vi "in_delta values.vi"(11 "x array":dbl[](array[numeric])) -> (3 "x delta values":dbl[](array[numeric]))   [LabVIEW 2020, in "NI_Gmath.lvlib"]
uses:
  NI_Gmath.lvlib
  NI_AALPro.lvlib
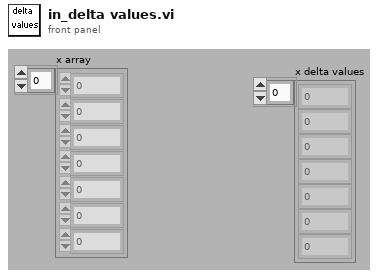
[diagram p1: front panel]
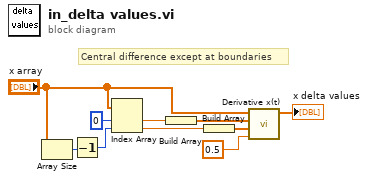
[diagram p0: block diagram]
diagram:
  # "Central difference except at boundaries"
  n1 = Array Size(array="x array") -> (size(s)=w10:i32)
  n2 = Decrement(x=w10) -> (x-1=w8:i32)
  n3 = Index Array(array="x array", index #1=0 ("index"), index #2=w8) -> (element #1=w7:dbl, element #2=w5:dbl)
  n4 = Build Array(w7) -> (w6:dbl[])
  n5 = Build Array(w5) -> (w4:dbl[])
  n6 = call "Derivative x(t).vi"("dt"=0.5, "Final Condition"=w4, "Initial Condition"=w6, "X"="x array") -> ("dX/dt"=→"x delta values":dbl[])  [unwired: 6 in, 1 out]
